vi "RFSW Set.vi"(6 "RFSW State":T1=enum."1", 7 "RFSW Letter":T2, 8 "error in (no error)":errorcluster, 11 "SN":string) -> (0 "error out":errorcluster, 1 "Model Name":string, 2 "Connected?":bool, 3 "Ref_Out":refnum<k24>)   [LabVIEW 2020]
uses:
  C:/Projects/Github/LabVIEW-Tools/Mini-Circuits-RF-Switch/DLL/mcl_RF_Switch_Controller64.dll
  DLL/mcl_RF_Switch_Controller64.dll
  RFSW Letter.ctl
  RFSW State.ctl
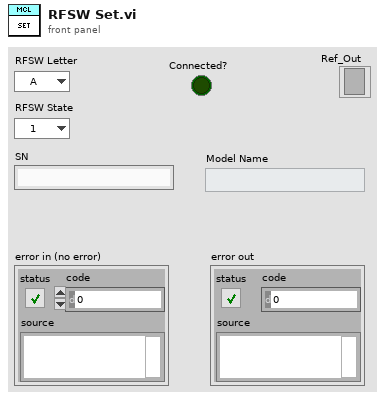
[diagram p1: front panel]
types:
  T1 = typedef "RFSW State.ctl" = enum16{"0", "1", "2", "3", "4", "5", "6"}
  T2 = typedef "RFSW Letter.ctl" = enum16{"A", "B"}
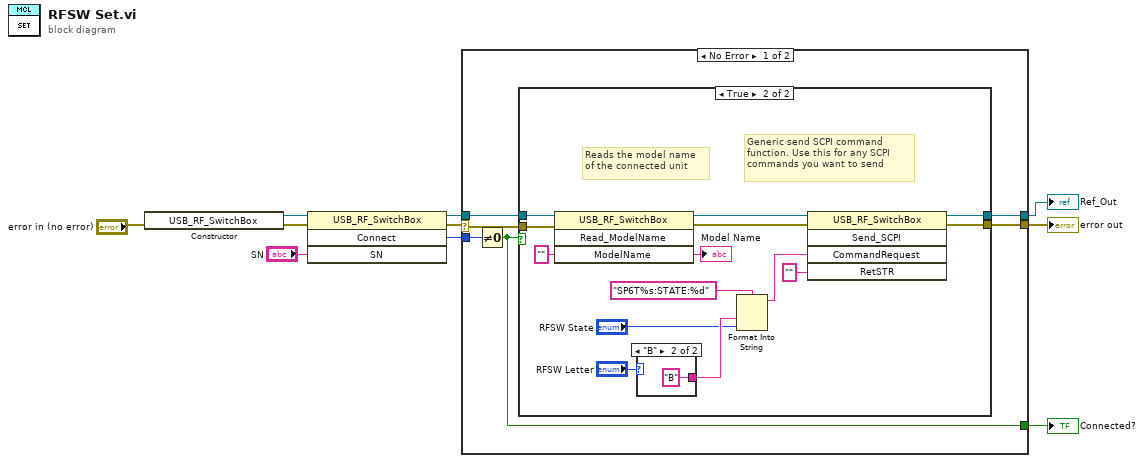
[diagram p0: block diagram]
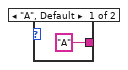
[diagram p3: hidden frame]
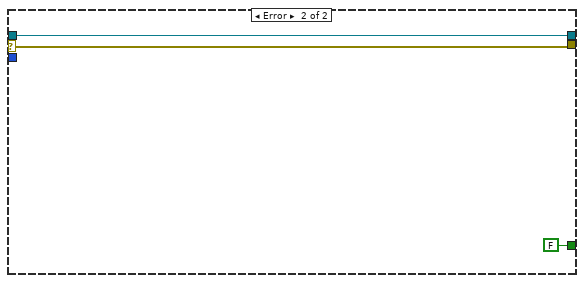
[diagram p4: hidden frame]
diagram:
  n1 = constructor class="USB_RF_SwitchBox"(error in="error in (no error)") -> (reference out=w4:refnum<k24>, error out=w5:errorcluster)  [unwired: 2 in, 1 out]
  n2 = invoke class="USB_RF_SwitchBox" method="Connect"(reference=w4, error in=w5, "SN"="SN") -> (reference out=w10:refnum<k24>, error out=w9:errorcluster, "Connect"=w8:i32)  [unwired: 1 in, 1 out]
  n3 = case shown="No Error" w9 {
    selector: w9 -> [w15 w37]
    tunnel: w10 -> [w16 w36]
    tunnel: w8 -> [w14 _]
    tunnel: [w13 w37] -> w7
    tunnel: [w12 w36] -> w2
    tunnel: [w11 FALSE] -> w1
    frame No Error {
      n4 = Not Equal To 0?(x=w14) -> (x != 0?=w11:bool)
      n5 = case shown="True" w11 {
        tunnel: w16 -> [w17 w27]
        tunnel: w15 -> [w18 w24]
        tunnel: [w18 w23] -> w13
        tunnel: [w17 w22] -> w12
        frame False {
        }
        frame True {
          # "Reads the model name of the connected unit"
          # "Generic send SCPI command function. Use this for any SCPI commands you want to send"
          n6 = invoke class="USB_RF_SwitchBox" method="Read_ModelName"(reference=w27, error in=w24, "ModelName"="") -> (reference out=w25:refnum<k24>, error out=w26:errorcluster, "ModelName"=→"Model Name":string)  [unwired: 1 in, 1 out]
          n7 = case shown="\"B\"" "RFSW Letter" {
            tunnel: ["A" "B"] -> w20
            frame "A", Default {
            }
            frame "B" {
            }
          }
          n8 = Format Into String(format string="SP6T%s:STATE:%d", w20, "RFSW State") -> (resulting string=w32:string)  [unwired: 2 in, 1 out]
          n9 = invoke class="USB_RF_SwitchBox" method="Send_SCPI"(reference=w25, error in=w26, "CommandRequest"=w32, "RetSTR"="") -> (reference out=w22:refnum<k24>, error out=w23:errorcluster)  [unwired: 1 in, 3 out]
        }
      }
    }
    frame Error {
    }
  }
  "error out" <- w7
  "Ref_Out" <- w2
  "Connected?" <- w1
